vi "Stepper Run Mode Example.vi"() -> ()   [LabVIEW 2012, in "Phidget Stepper.lvlib"]
uses:
  <instrlib>/Phidgets/Phidget Stepper/Phidget Stepper.lvlib
  <instrlib>/Phidgets/Phidget Stepper/Public/StepperStart.vi
  <instrlib>/Phidgets/Phidget Stepper/Public/StepperClose.vi
  <instrlib>/Phidgets/Phidget Common/Phidget Common.lvlib
panel:
  in  "Stepper Initialization Data":T1={"Control Mode"=1, " Rescale Factor"=1.0, "Velocity Limit"=0.0, "Acceleration"=10000.0, "Current Limit"=1.0} {"Control Mode" items=["Step", "Run"]}
  in  "Velocity Limit":dbl
  in  "stop":bool
  out "Velocity":dbl
  out "Position":dbl
  out "Moving":bool
  in  "Device Info":T2={"Serial Number"=-1, "Channel"=0, "Port"=0}
  out "Attached?":bool
  out "Serial Number Return":i32
  out "error out":errorcluster
  # "NOTE: The default\nVelocity Limit and\nAcceleration\nparameters will not\nwork with the 1062.\nThese may be\nboth set to 200\n(or any other value \nin the valid range)\nfor the device to\nwork."
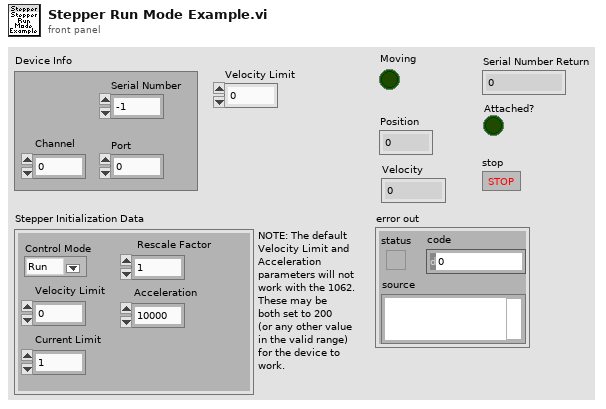
[diagram p1: front panel]
types:
  T1 = cluster{"Control Mode":u16, " Rescale Factor":dbl, "Velocity Limit":dbl, "Acceleration":dbl, "Current Limit":dbl}
  T2 = cluster{"Serial Number":i32, "Channel":i32, "Port":i32}
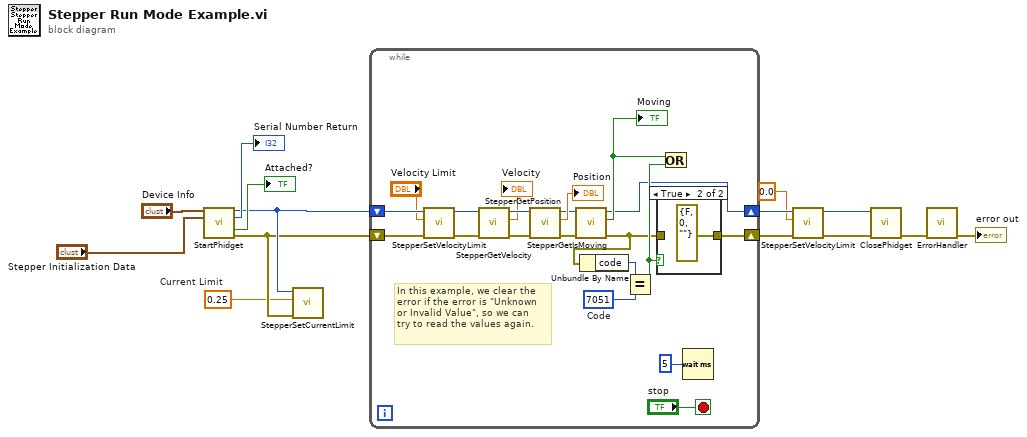
[diagram p0: block diagram]
diagram:
  w1 = 0.25  # Current Limit
  n1 = call-poly <instrlib>:"StartPhidget.vi"("Device Info"="Device Info", "Stepper Initialization Data"="Stepper Initialization Data") -> ("Phidget ID"=w3:u64, "Serial Number Return"=→"Serial Number Return":i32, "Attached?"=→"Attached?":bool, "error out"=w2:errorcluster)  [unwired: 10 in]
  n2 = call <instrlib>:"StepperSetCurrentLimit.vi"("error in (no error)"=w2, "Current Limit"=w1, "Device In"=w3) -> ()  [unwired: 6 in, 2 out]
  n3 = while {
    shift-right: [w19] -> w10
    shift-left: w3 -> [w26]
    shift-right: [w16] -> w9
    shift-left: w2 -> [w25]
    stop <- "stop" stop-if-true
    w22 = 7051  # Code
    # "In this example, we clear the\nerror if the error is \"Unknown\nor Invalid Value\", so we can\ntry to read the values again."
    n4 = call <instrlib>:"StepperSetVelocityLimit.vi"("error in (no error)"=w25, "Velocity Limit"="Velocity Limit", "Device In"=w26) -> ("error out"=w28:errorcluster, "Device Out"=w27:u64)  [unwired: 6 in]
    n5 = call <instrlib>:"StepperGetVelocity.vi"("error in (no error)"=w28, "Device In"=w27) -> ("error out"=w32:errorcluster, "Velocity"=→"Velocity":dbl, "Device Out"=w31:u64)  [unwired: 6 in]
    n6 = call <instrlib>:"StepperGetPosition.vi"("error in (no error)"=w32, "Device In"=w31) -> ("error out"=w18:errorcluster, "Position"=→"Position":dbl, "Device Out"=w17:u64)  [unwired: 6 in]
    n7 = call <instrlib>:"StepperGetIsMoving.vi"("error in (no error)"=w18, "Device In"=w17) -> ("error out"=w15:errorcluster, "Moving"=w20:bool, "Device Out"=w19:u64)  [unwired: 6 in]
    "Moving" <- w20
    n8 = Unbundle By Name(w15) -> ("code"=w23:i32)
    n9 = Equal?(x=w23, y=w22) -> (x = y?=w21:bool)
    n10 = case shown="True" w21 {
      tunnel: w15 -> [w35 _]
      tunnel: [w35 errorcluster {"status"=FALSE, "code"=0, "source"=""} ("error constant")] -> w16
      frame False {
      }
      frame True {
      }
    }
    n11 = Or(x=w20, y=w21) -> ()  [unwired: 1 out]
    n12 = Wait (ms)(milliseconds to wait=u32 5) -> ()  [unwired: 1 out]
  }
  n13 = call <instrlib>:"StepperSetVelocityLimit.vi"("error in (no error)"=w9, "Velocity Limit"=0.0, "Device In"=w10) -> ("error out"=w8:errorcluster, "Device Out"=w7:u64)  [unwired: 6 in]
  n14 = call-poly <instrlib>:"ClosePhidget.vi"("error in"=w8, "Device In"=w7) -> ("error out"=w14:errorcluster)  [unwired: 9 in]
  n15 = call <instrlib>:"ErrorHandler.vi"("error in"=w14) -> ("error out"=→"error out":errorcluster)  [unwired: 9 in, 1 out]
